vi "星际大战完整版.vi"() -> ()   [LabVIEW 2018]
panel:
  in  "关卡":dbl
  out "失败界面":picture
  out "胜利界面":picture
  out "敌机是否入侵":bool
  out "得分":dbl
  out "战舰爆炸":picture
  out "血量":dbl
  out "战舰血量":T1 scale=0.0..100.0
  out "敌机爆炸":picture
  in  "敌机数量":dbl
  in  "敌机速度":dbl
  out "敌机":picture
  out "按键":dbl
  out "战舰":T2
  out "激光武器1":T3
  out "激光武器 2":T3
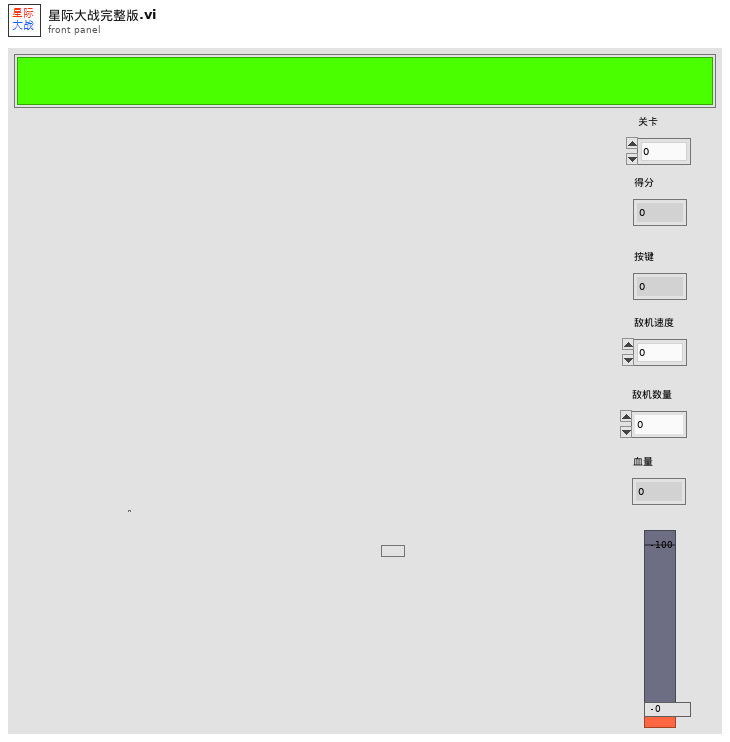
[diagram p1: front panel]
types:
  T1 = typedef "战列巡洋舰_血条.ctl" = dbl
  T2 = typedef "战列巡洋舰.ctl" = picture
  T3 = typedef "战列巡洋舰_激光武器.ctl" = picture
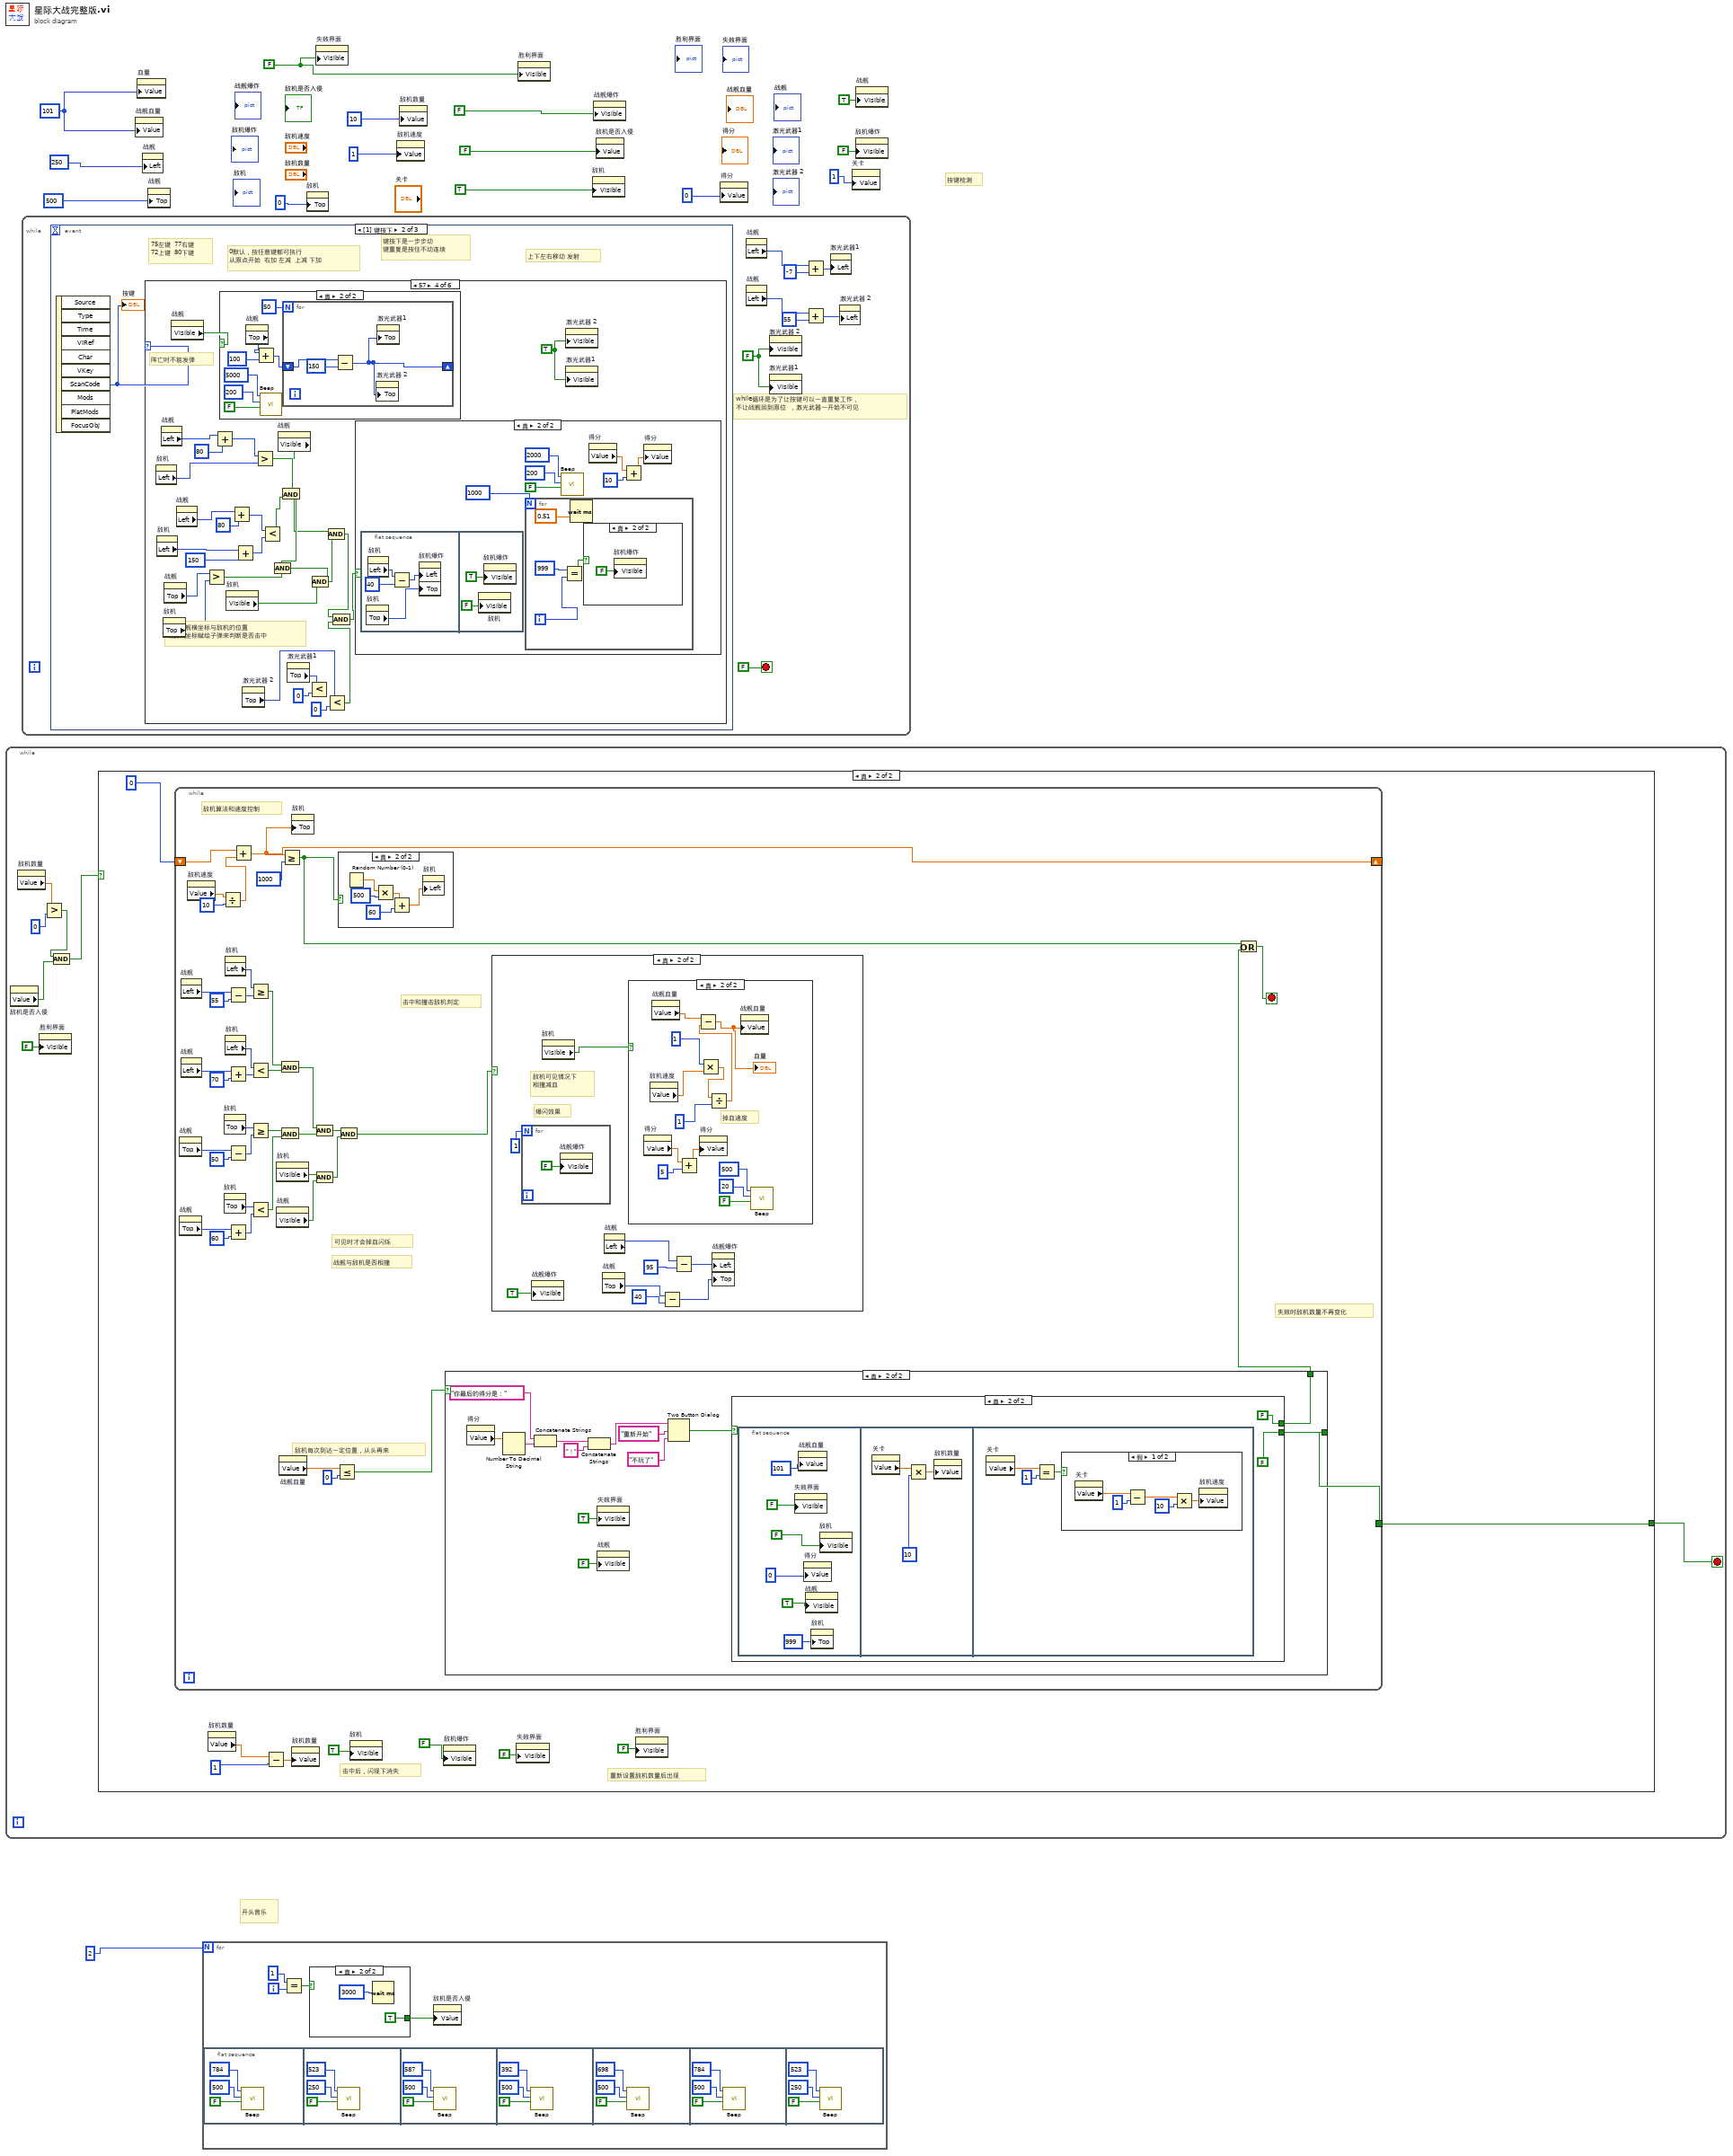
[diagram p0: block diagram]
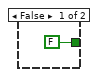
[diagram p2: hidden frame]
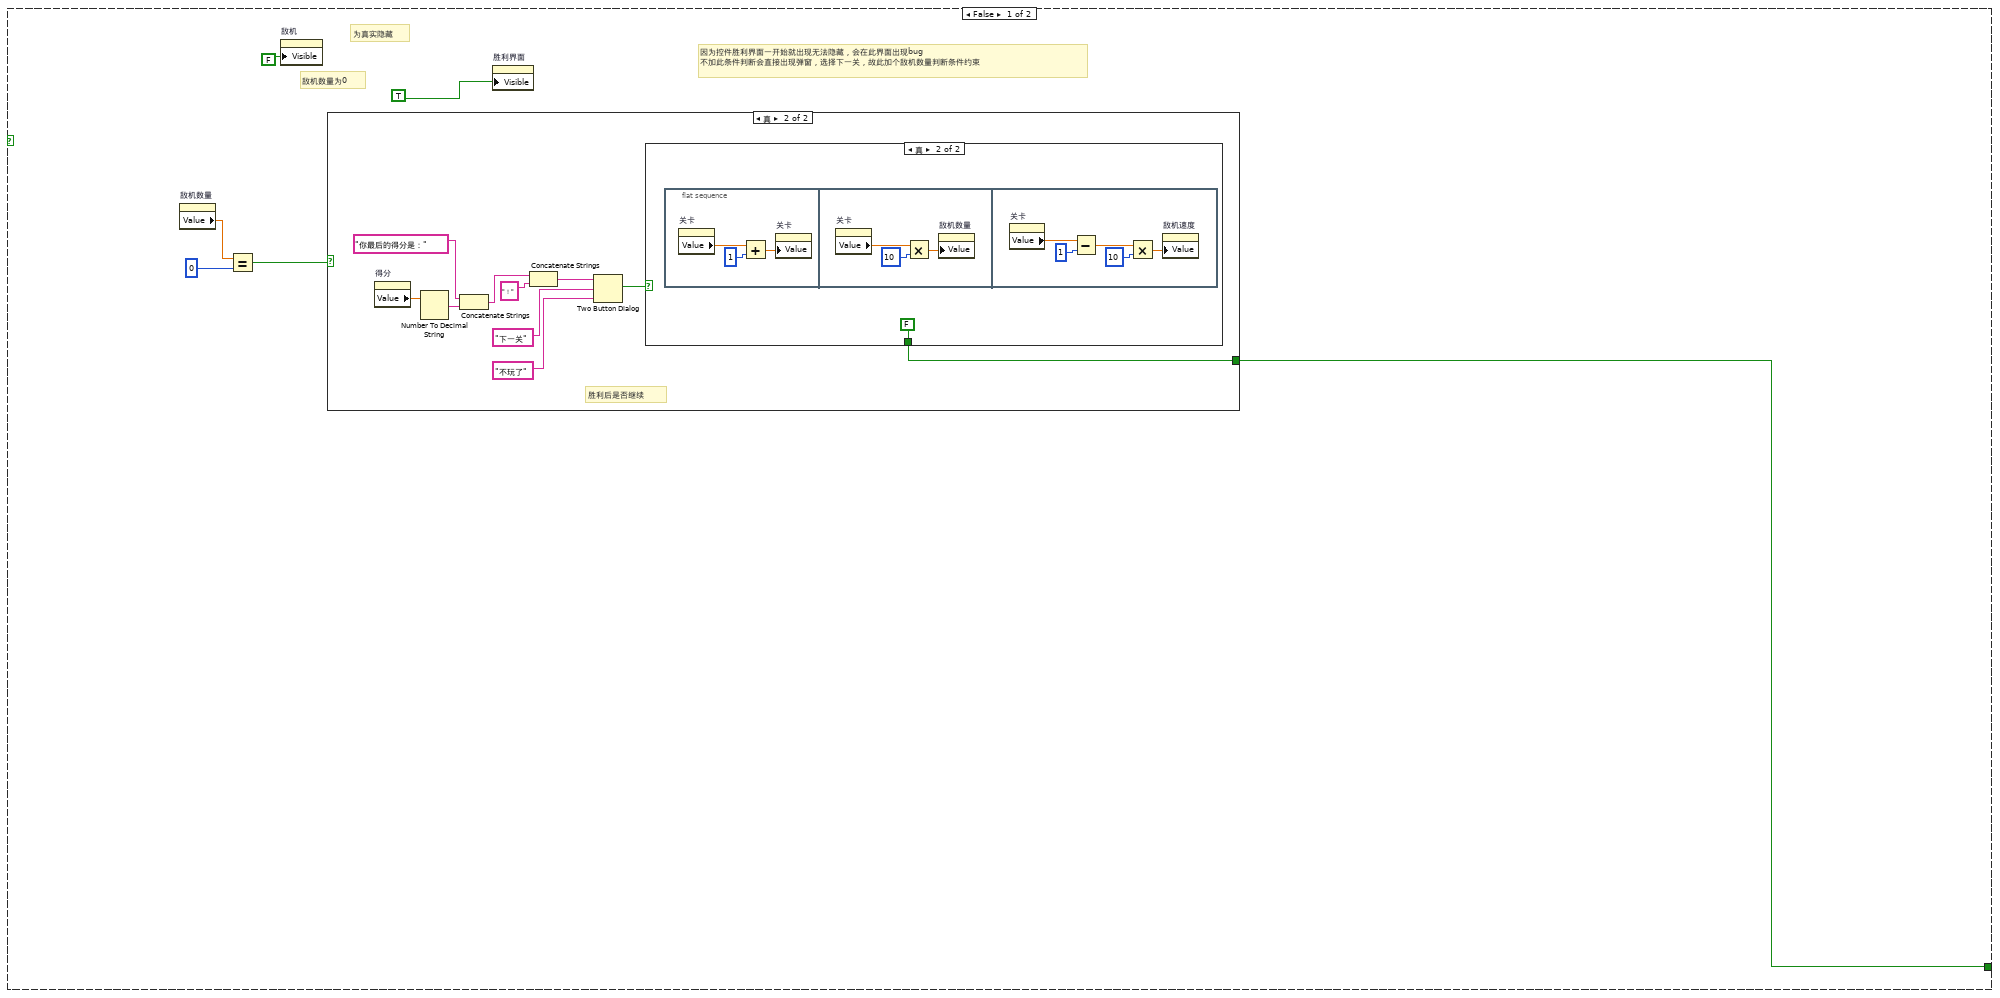
[diagram p3: hidden frame]
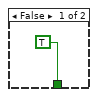
[diagram p5: hidden frame]
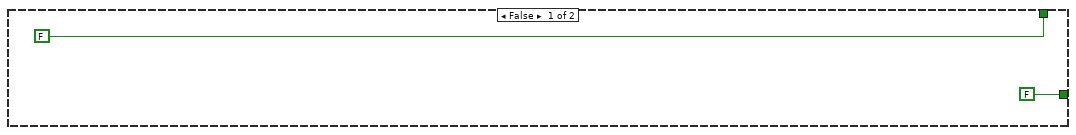
[diagram p6: hidden frame]
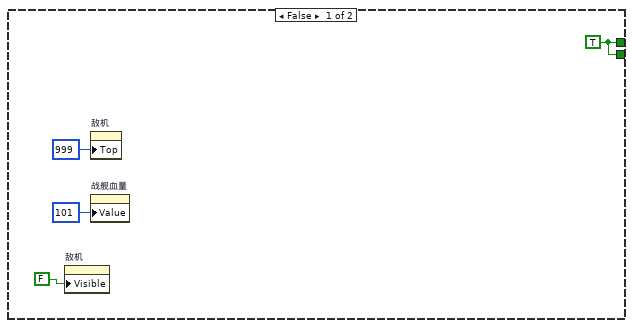
[diagram p7: hidden frame]
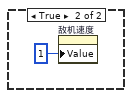
[diagram p8: hidden frame]
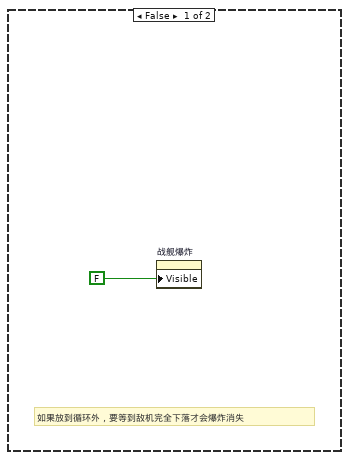
[diagram p9: hidden frame]
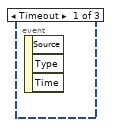
[diagram p12: hidden frame]
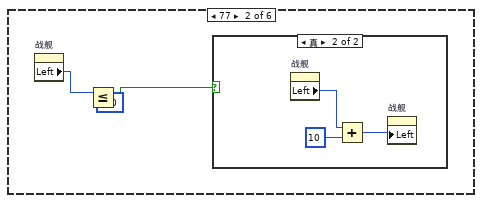
[diagram p14: hidden frame]
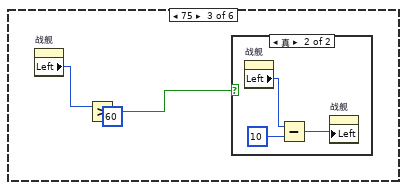
[diagram p16: hidden frame]
diagram:
  w1 = FALSE ("可见")
  w9 = 101
  # "开头音乐"
  # "按键检测"
  n1 = while {
    stop <- w17 stop-if-true
    n2 = property on="敌机是否入侵" class="Bool (严格)"() -> ("Value"=w20:bool)  [unwired: 2 in, 2 out]
    n3 = property on="敌机数量" class="DigNum (严格)"() -> ("Value"=w22:dbl)  [unwired: 2 in, 2 out]
    n4 = property on="胜利界面" class="Pict"("Visible"=FALSE ("可见")) -> ()  [unwired: 2 in, 2 out]
    n5 = Greater?(x=w22, y=0) -> (0:w19:bool)
    n6 = And(x=w19, y=w20) -> (x .and. y?=w18:bool)
    n7 = case shown="真" w18 {
      tunnel: [w26 w53] -> w17
      frame False {
        # "因为控件胜利界面一开始就出现无法隐藏，会在此界面出现bug\n不加此条件判断会直接出现弹窗，选择下一关，故此加个敌机数量判断条件约束"
        # "敌机数量为0"
        # "为真实隐藏"
        n8 = property on="敌机数量" class="DigNum (严格)"() -> ("Value"=w25:dbl)  [unwired: 2 in, 2 out]
        n9 = Equal?(x=w25, y=0) -> (x = y?=w23:bool)
        n10 = property on="敌机" class="Pict"("Visible"=FALSE ("可见")) -> ()  [unwired: 2 in, 2 out]
        n11 = case shown="真" w23 {
          tunnel: [_ w29] -> w26
          frame False {
          }
          frame True {
            # "胜利后是否继续"
            n12 = property on="得分" class="DigNum (严格)"() -> ("Value"=w37:dbl)  [unwired: 2 in, 2 out]
            n13 = Number To Decimal String(number=w37) -> (decimal integer string=w35:string)  [unwired: 1 in]
            n14 = Concatenate Strings("你最后的得分是：", w35) -> (w34:string)
            n15 = Concatenate Strings(w34, "！") -> (w32:string)
            n16 = Two Button Dialog(message=w32, 1:"不玩了" ("F按钮名称（“取消”）"), 2:"下一关" ("T按钮名称（“确定”）")) -> (T button?=w38:bool)
            n17 = case shown="真" w38 {
              tunnel: [TRUE FALSE] -> w29
              frame False {
              }
              frame True {
                n18 = flat-sequence {
                  frame #0 {
                    n19 = property on="关卡" class="DigNum (严格)"() -> ("Value"=w43:dbl)  [unwired: 2 in, 2 out]
                    n20 = Add(x=w43, y=1) -> (x+y=w41:dbl)
                    n21 = property on="关卡" class="DigNum (严格)"("Value"=w41) -> ()  [unwired: 2 in, 2 out]
                  }
                  frame #1 {
                    n22 = property on="关卡" class="DigNum (严格)"() -> ("Value"=w45:dbl)  [unwired: 2 in, 2 out]
                    n23 = Multiply(x=w45, y=10) -> (x*y=w46:dbl)
                    n24 = property on="敌机数量" class="DigNum (严格)"("Value"=w46) -> ()  [unwired: 2 in, 2 out]
                  }
                  frame #2 {
                    n25 = property on="关卡" class="DigNum (严格)"() -> ("Value"=w50:dbl)  [unwired: 2 in, 2 out]
                    n26 = Subtract(x=w50, y=1) -> (x-y=w48:dbl)
                    n27 = Multiply(x=w48, y=10) -> (x*y=w47:dbl)
                    n28 = property on="敌机速度" class="DigNum (严格)"("Value"=w47) -> ()  [unwired: 2 in, 2 out]
                  }
                }
              }
            }
          }
        }
        n29 = property on="胜利界面" class="Pict"("Visible"=TRUE ("可见")) -> ()  [unwired: 2 in, 2 out]
      }
      frame True {
        # "重新设置敌机数量后出现"
        # "击中后，闪现下消失"
        # "敌机每次到达一定位置，从头再来"
        n30 = while {
          shift-right: [w98] -> _
          shift-left: 0 -> [w100]
          tunnel: [w64] -> w53
          stop <- w62 stop-if-true
          # "失败时敌机数量不再变化"
          # "击中和撞击敌机判定"
          # "可见时才会掉血闪烁"
          # "战舰与敌机是否相撞"
          # "敌机算法和速度控制"
          n31 = property on="战舰" class="Pict (严格)"() -> ("Top"=w83:i32)  [unwired: 2 in, 2 out]
          n32 = property on="战舰" class="Pict (严格)"() -> ("Top"=w77:i32)  [unwired: 2 in, 2 out]
          n33 = property on="战舰" class="Pict (严格)"() -> ("Left"=w93:i32)  [unwired: 2 in, 2 out]
          n34 = property on="战舰" class="Pict (严格)"() -> ("Left"=w87:i32)  [unwired: 2 in, 2 out]
          n35 = property on="敌机速度" class="DigNum (严格)"() -> ("Value"=w97:dbl)  [unwired: 2 in, 2 out]
          n36 = Divide(x=w97, y=10) -> (x/y=w96:dbl)
          n37 = property on="敌机" class="Pict"() -> ("Top"=w84:i32)  [unwired: 2 in, 2 out]
          n38 = property on="敌机" class="Pict"() -> ("Top"=w76:i32)  [unwired: 2 in, 2 out]
          n39 = property on="敌机" class="Pict"() -> ("Left"=w94:i32)  [unwired: 2 in, 2 out]
          n40 = property on="敌机" class="Pict"() -> ("Left"=w89:i32)  [unwired: 2 in, 2 out]
          n41 = Subtract(x=w93, y=55) -> (x-y=w92:i32)
          n42 = Add(x=w87, y=70) -> (x+y=w86:i32)
          n43 = Subtract(x=w83, y=50) -> (x-y=w81:i32)
          n44 = Add(x=w77, y=60) -> (x+y=w79:i32)
          n45 = Add(x=w100, y=w96) -> (x+y=w98:dbl)
          n46 = Greater Or Equal?(x=w94, y=w92) -> (x >= y?=w90:bool)
          n47 = Less?(x=w89, y=w86) -> (x < y?=w85:bool)
          n48 = Greater Or Equal?(x=w84, y=w81) -> (x >= y?=w75:bool)
          n49 = Less?(x=w76, y=w79) -> (x < y?=w74:bool)
          n50 = property on="敌机" class="Pict"() -> ("Visible"=w67:bool)  [unwired: 2 in, 2 out]
          n51 = property on="战舰" class="Pict (严格)"() -> ("Visible"=w66:bool)  [unwired: 2 in, 2 out]
          n52 = And(x=w90, y=w85) -> (x .and. y?=w80:bool)
          n53 = And(x=w75, y=w74) -> (x .and. y?=w73:bool)
          n54 = property on="战舰血量" class="Slide (严格)"() -> ("Value"=w69:T1)  [unwired: 2 in, 2 out]
          n55 = Greater Or Equal?(x=w98, y=1000) -> (x >= y?=w63:bool)
          n56 = property on="敌机" class="Pict"("Top"=w98) -> ()  [unwired: 2 in, 2 out]
          n57 = And(x=w80, y=w73) -> (x .and. y?=w72:bool)
          n58 = And(x=w67, y=w66) -> (x .and. y?=w65:bool)
          n59 = Less Or Equal?(x=w69, y=0) -> (x <= y?=w70:bool)
          n60 = case shown="真" w63 {
            frame False {
            }
            frame True {
              n61 = Random Number (0-1)() -> (number: 0 to 1=w168:dbl)
              n62 = Multiply(x=w168, y=500) -> (x*y=w166:dbl)
              n63 = Add(x=w166, y=60) -> (x+y=w165:dbl)
              n64 = property on="敌机" class="Pict"("Left"=w165) -> ()  [unwired: 2 in, 2 out]
            }
          }
          n65 = And(x=w72, y=w65) -> (x .and. y?=w71:bool)
          n66 = case shown="真" w70 {
            tunnel: [FALSE w104] -> w64
            tunnel: [FALSE w103] -> w61
            frame False {
            }
            frame True {
              n67 = property on="得分" class="DigNum (严格)"() -> ("Value"=w115:dbl)  [unwired: 2 in, 2 out]
              n68 = Number To Decimal String(number=w115) -> (decimal integer string=w114:string)  [unwired: 1 in]
              n69 = Concatenate Strings("你最后的得分是：", w114) -> (w113:string)
              n70 = Concatenate Strings(w113, "！") -> (w112:string)
              n71 = property on="失败界面" class="Pict"("Visible"=TRUE ("可见")) -> ()  [unwired: 2 in, 2 out]
              n72 = property on="战舰" class="Pict (严格)"("Visible"=FALSE ("可见")) -> ()  [unwired: 2 in, 2 out]
              n73 = Two Button Dialog(message=w112, 1:"不玩了" ("F按钮名称（“取消”）"), 2:"重新开始" ("T按钮名称（“确定”）")) -> (T button?=w107:bool)
              n74 = case shown="真" w107 {
                tunnel: [w117 FALSE] -> w104
                tunnel: [w117 FALSE] -> w103
                frame False {
                  w117 = TRUE
                  n75 = property on="敌机" class="Pict"("Visible"=FALSE ("可见")) -> ()  [unwired: 2 in, 2 out]
                  n76 = property on="敌机" class="Pict"("Top"=999 ("位置:置顶")) -> ()  [unwired: 2 in, 2 out]
                  n77 = property on="战舰血量" class="Slide (严格)"("Value"=101) -> ()  [unwired: 2 in, 2 out]
                }
                frame True {
                  n78 = flat-sequence {
                    frame #0 {
                      n79 = property on="失败界面" class="Pict"("Visible"=FALSE ("可见")) -> ()  [unwired: 2 in, 2 out]
                      n80 = property on="战舰血量" class="Slide (严格)"("Value"=101) -> ()  [unwired: 2 in, 2 out]
                      n81 = property on="得分" class="DigNum (严格)"("Value"=0) -> ()  [unwired: 2 in, 2 out]
                      n82 = property on="战舰" class="Pict (严格)"("Visible"=TRUE ("可见")) -> ()  [unwired: 2 in, 2 out]
                      n83 = property on="敌机" class="Pict"("Top"=999 ("位置:置顶")) -> ()  [unwired: 2 in, 2 out]
                      n84 = property on="敌机" class="Pict"("Visible"=FALSE ("可见")) -> ()  [unwired: 2 in, 2 out]
                    }
                    frame #1 {
                      n85 = property on="关卡" class="DigNum (严格)"() -> ("Value"=w128:dbl)  [unwired: 2 in, 2 out]
                      n86 = Multiply(x=w128, y=10) -> (x*y=w130:dbl)
                      n87 = property on="敌机数量" class="DigNum (严格)"("Value"=w130) -> ()  [unwired: 2 in, 2 out]
                    }
                    frame #2 {
                      n88 = property on="关卡" class="DigNum (严格)"() -> ("Value"=w133:dbl)  [unwired: 2 in, 2 out]
                      n89 = Equal?(x=w133, y=1) -> (x = y?=w131:bool)
                      n90 = case shown="假" w131 {
                        frame False {
                          n91 = property on="关卡" class="DigNum (严格)"() -> ("Value"=w137:dbl)  [unwired: 2 in, 2 out]
                          n92 = Subtract(x=w137, y=1) -> (x-y=w134:dbl)
                          n93 = Multiply(x=w134, y=10) -> (x*y=w138:dbl)
                          n94 = property on="敌机速度" class="DigNum (严格)"("Value"=w138) -> ()  [unwired: 2 in, 2 out]
                        }
                        frame True {
                          n95 = property on="敌机速度" class="DigNum (严格)"("Value"=1) -> ()  [unwired: 2 in, 2 out]
                        }
                      }
                    }
                  }
                }
              }
            }
          }
          n96 = case shown="真" w71 {
            frame False {
              # "如果放到循环外，要等到敌机完全下落才会爆炸消失"
              n97 = property on="战舰爆炸" class="Pict"("Visible"=FALSE ("可见")) -> ()  [unwired: 2 in, 2 out]
            }
            frame True {
              # "爆闪效果"
              # "敌机可见情况下\n相撞减血"
              n98 = for {
                N: 1 -> [_]
                n99 = property on="战舰爆炸" class="Pict"("Visible"=FALSE ("可见")) -> ()  [unwired: 2 in, 2 out]
              }
              n100 = property on="战舰爆炸" class="Pict"("Visible"=TRUE ("可见")) -> ()  [unwired: 2 in, 2 out]
              n101 = property on="敌机" class="Pict"() -> ("Visible"=w149:bool)  [unwired: 2 in, 2 out]
              n102 = property on="战舰" class="Pict (严格)"() -> ("Top"=w144:i32)  [unwired: 2 in, 2 out]
              n103 = property on="战舰" class="Pict (严格)"() -> ("Left"=w147:i32)  [unwired: 2 in, 2 out]
              n104 = case shown="真" w149 {
                frame False {
                }
                frame True {
                  # "掉血速度"
                  n105 = property on="得分" class="DigNum (严格)"() -> ("Value"=w156:dbl)  [unwired: 2 in, 2 out]
                  n106 = property on="敌机速度" class="DigNum (严格)"() -> ("Value"=w162:dbl)  [unwired: 2 in, 2 out]
                  n107 = property on="战舰血量" class="Slide (严格)"() -> ("Value"=w163:T1)  [unwired: 2 in, 2 out]
                  n108 = Add(x=w156, y=5) -> (x+y=w155:dbl)
                  n109 = Multiply(x=1, y=w162) -> (x*y=w161:dbl)
                  n110 = property on="得分" class="DigNum (严格)"("Value"=w155) -> ()  [unwired: 2 in, 2 out]
                  n111 = Divide(x=w161, y=1) -> (x/y=w158:dbl)
                  n112 = Subtract(x=w163, y=w158) -> (x-y=w157:T1)
                  "血量" <- w157
                  n113 = property on="战舰血量" class="Slide (严格)"("Value"=w157) -> ()  [unwired: 2 in, 2 out]
                  n114 = call <vilib>:"Beep.vi"("use system alert? (T)"=FALSE, "duration (msec)"=u32 20, "frequency (Hz)"=u32 500) -> ()  [unwired: 9 in]
                }
              }
              n115 = Subtract(x=w144, y=40) -> (x-y=w142:i32)
              n116 = Subtract(x=w147, y=95) -> (x-y=w145:i32)
              n117 = property on="战舰爆炸" class="Pict"("Left"=w145, "Top"=w142) -> ()  [unwired: 2 in, 2 out]
            }
          }
          n118 = Or(x=w63, y=w61) -> (x .or. y?=w62:bool)
        }
        n119 = property on="敌机数量" class="DigNum (严格)"() -> ("Value"=w58:dbl)  [unwired: 2 in, 2 out]
        n120 = Subtract(x=w58, y=1) -> (x-y=w59:dbl)
        n121 = property on="敌机数量" class="DigNum (严格)"("Value"=w59) -> ()  [unwired: 2 in, 2 out]
        n122 = property on="敌机" class="Pict"("Visible"=TRUE ("可见")) -> ()  [unwired: 2 in, 2 out]
        n123 = property on="敌机爆炸" class="Pict"("Visible"=FALSE ("可见")) -> ()  [unwired: 2 in, 2 out]
        n124 = property on="失败界面" class="Pict"("Visible"=FALSE ("可见")) -> ()  [unwired: 2 in, 2 out]
        n125 = property on="胜利界面" class="Pict"("Visible"=FALSE ("可见")) -> ()  [unwired: 2 in, 2 out]
      }
    }
  }
  n126 = while {
    stop <- FALSE stop-if-true
    w169 = FALSE
    # "while循环是为了让按键可以一直重复工作，\n不让战舰回到原位  ，激光武器一开始不可见"
    n127 = event shown="[1] 键按下" {
      selector: _ -> [_ _ _]
      dyn-events: _ -> [_ _ _]
      timeout: _ -> [_ _ _]
      event Timeout {
        n128 = event-data() -> ()  [unwired: 1 in, 3 out]
      }
      event Key Down {
        # "上下左右移动 发射"
        # "键按下是一步步动\n键重复是按住不动连续"
        # "75左键  77右键\n72上键  80下键"
        # "0默认，按任意键都可执行\n从原点开始  右加 左减  上减 下加"
        n129 = event-data() -> ("ScanCode"=w177:i16)  [unwired: 1 in, 9 out]
        "按键" <- w177
        n130 = case shown="57" w177 {
          frame 0, Default {
          }
          frame 77 {
            n131 = property on="战舰" class="Pict (严格)"() -> ("Left"=w180:i32)  [unwired: 2 in, 2 out]
            n132 = Less Or Equal?(x=w180, y=500) -> (x <= y?=w178:bool)
            n133 = case shown="真" w178 {
              frame False {
              }
              frame True {
                n134 = property on="战舰" class="Pict (严格)"() -> ("Left"=w182:i32)  [unwired: 2 in, 2 out]
                n135 = Add(x=w182, y=10) -> (x+y=w183:i32)
                n136 = property on="战舰" class="Pict (严格)"("Left"=w183) -> ()  [unwired: 2 in, 2 out]
              }
            }
          }
          frame 75 {
            n137 = property on="战舰" class="Pict (严格)"() -> ("Left"=w186:i32)  [unwired: 2 in, 2 out]
            n138 = Greater?(x=w186, y=60) -> (0:w184:bool)
            n139 = case shown="真" w184 {
              frame False {
              }
              frame True {
                n140 = property on="战舰" class="Pict (严格)"() -> ("Left"=w188:i32)  [unwired: 2 in, 2 out]
                n141 = Subtract(x=w188, y=10) -> (x-y=w189:i32)
                n142 = property on="战舰" class="Pict (严格)"("Left"=w189) -> ()  [unwired: 2 in, 2 out]
              }
            }
          }
          frame 57 {
            w218 = TRUE
            # "阵亡时不能发弹"
            # "判断战舰横坐标与敌机的位置\n战舰纵坐标赋给子弹来判断是否击中"
            n143 = property on="敌机" class="Pict"() -> ("Left"=w215:i32)  [unwired: 2 in, 2 out]
            n144 = property on="敌机" class="Pict"() -> ("Left"=w208:i32)  [unwired: 2 in, 2 out]
            n145 = property on="战舰" class="Pict (严格)"() -> ("Left"=w217:i32)  [unwired: 2 in, 2 out]
            n146 = property on="敌机" class="Pict"() -> ("Top"=w202:i32)  [unwired: 2 in, 2 out]
            n147 = property on="战舰" class="Pict (严格)"() -> ("Top"=w203:i32)  [unwired: 2 in, 2 out]
            n148 = property on="战舰" class="Pict (严格)"() -> ("Visible"=w197:bool)  [unwired: 2 in, 2 out]
            n149 = property on="战舰" class="Pict (严格)"() -> ("Left"=w210:i32)  [unwired: 2 in, 2 out]
            n150 = Greater?(x=w203, y=w202) -> (0:w204:bool)
            n151 = Add(x=w217, y=80) -> (x+y=w214:i32)
            n152 = case shown="真" w197 {
              frame False {
              }
              frame True {
                n153 = property on="战舰" class="Pict (严格)"() -> ("Top"=w224:i32)  [unwired: 2 in, 2 out]
                n154 = Add(x=w224, y=100) -> (x+y=w222:i32)
                n155 = call <vilib>:"Beep.vi"("use system alert? (T)"=FALSE, "duration (msec)"=u32 200, "frequency (Hz)"=u32 5000) -> ()  [unwired: 9 in]
                n156 = for {
                  N: 50 -> [_]
                  shift-right: [w226] -> _
                  shift-left: w222 -> [w228]
                  n157 = Subtract(x=w228, y=150) -> (x-y=w226:i32)
                  n158 = property on="激光武器 2" class="Pict (严格)"("Top"=w226) -> ()  [unwired: 2 in, 2 out]
                  n159 = property on="激光武器1" class="Pict (严格)"("Top"=w226) -> ()  [unwired: 2 in, 2 out]
                }
              }
            }
            n160 = property on="敌机" class="Pict"() -> ("Visible"=w200:bool)  [unwired: 2 in, 2 out]
            n161 = Add(x=w210, y=80) -> (x+y=w212:i32)
            n162 = Add(x=w208, y=150) -> (x+y=w207:i32)
            n163 = property on="激光武器 2" class="Pict (严格)"() -> ("Top"=w193:i32)  [unwired: 2 in, 2 out]
            n164 = Greater?(x=w214, y=w215) -> (0:w213:bool)
            n165 = Less?(x=w212, y=w207) -> (x < y?=w209:bool)
            n166 = property on="战舰" class="Pict (严格)"() -> ("Visible"=w199:bool)  [unwired: 2 in, 2 out]
            n167 = And(x=w213, y=w209) -> (x .and. y?=w205:bool)
            n168 = And(x=w205, y=w204) -> (x .and. y?=w201:bool)
            n169 = property on="激光武器1" class="Pict (严格)"() -> ("Top"=w195:i32)  [unwired: 2 in, 2 out]
            n170 = Less?(x=w195, y=0) -> ()  [unwired: 1 out]
            n171 = And(x=w201, y=w200) -> (x .and. y?=w198:bool)
            n172 = And(x=w199, y=w198) -> (x .and. y?=w191:bool)
            n173 = Less?(x=w193, y=0) -> (x < y?=w192:bool)
            n174 = And(x=w191, y=w192) -> (x .and. y?=w190:bool)
            n175 = case shown="真" w190 {
              frame False {
              }
              frame True {
                n176 = flat-sequence {
                  frame #0 {
                    n177 = property on="敌机" class="Pict"() -> ("Top"=w239:i32)  [unwired: 2 in, 2 out]
                    n178 = property on="敌机" class="Pict"() -> ("Left"=w237:i32)  [unwired: 2 in, 2 out]
                    n179 = Subtract(x=w237, y=40) -> (x-y=w236:i32)
                    n180 = property on="敌机爆炸" class="Pict"("Left"=w236, "Top"=w239) -> ()  [unwired: 2 in, 2 out]
                  }
                  frame #1 {
                    n181 = property on="敌机" class="Pict"("Visible"=FALSE ("可见")) -> ()  [unwired: 2 in, 2 out]
                    n182 = property on="敌机爆炸" class="Pict"("Visible"=TRUE ("可见")) -> ()  [unwired: 2 in, 2 out]
                  }
                }
                n183 = for {
                  N: 1000 -> [_]
                  i -> [w244]
                  n184 = Equal?(x=999, y=w244) -> (x = y?=w245:bool)
                  n185 = Wait (ms)(milliseconds to wait=0.51) -> ()  [unwired: 1 out]
                  n186 = case shown="真" w245 {
                    frame False {
                    }
                    frame True {
                      n187 = property on="敌机爆炸" class="Pict"("Visible"=FALSE ("可见")) -> ()  [unwired: 2 in, 2 out]
                    }
                  }
                }
                n188 = call <vilib>:"Beep.vi"("use system alert? (T)"=FALSE, "duration (msec)"=u32 200, "frequency (Hz)"=u32 2000) -> ()  [unwired: 9 in]
                n189 = property on="得分" class="DigNum (严格)"() -> ("Value"=w234:dbl)  [unwired: 2 in, 2 out]
                n190 = Add(x=w234, y=10) -> (x+y=w232:dbl)
                n191 = property on="得分" class="DigNum (严格)"("Value"=w232) -> ()  [unwired: 2 in, 2 out]
              }
            }
            n192 = property on="激光武器 2" class="Pict (严格)"("Visible"=w218) -> ()  [unwired: 2 in, 2 out]
            n193 = property on="激光武器1" class="Pict (严格)"("Visible"=w218) -> ()  [unwired: 2 in, 2 out]
          }
          frame 80 {
            n194 = property on="战舰" class="Pict (严格)"() -> ("Top"=w249:i32)  [unwired: 2 in, 2 out]
            n195 = Less?(x=w249, y=525) -> (x < y?=w247:bool)
            n196 = case shown="真" w247 {
              frame False {
              }
              frame True {
                n197 = property on="战舰" class="Pict (严格)"() -> ("Top"=w251:i32)  [unwired: 2 in, 2 out]
                n198 = Add(x=w251, y=10) -> (x+y=w250:i32)
                n199 = property on="战舰" class="Pict (严格)"("Top"=w250) -> ()  [unwired: 2 in, 2 out]
              }
            }
          }
          frame 72 {
            n200 = property on="战舰" class="Pict (严格)"() -> ("Top"=w255:i32)  [unwired: 2 in, 2 out]
            n201 = Greater Or Equal?(x=w255, y=25) -> (x >= y?=w254:bool)
            n202 = case shown="真" w254 {
              frame False {
              }
              frame True {
                n203 = property on="战舰" class="Pict (严格)"() -> ("Top"=w258:i32)  [unwired: 2 in, 2 out]
                n204 = Subtract(x=w258, y=10) -> (x-y=w257:i32)
                n205 = property on="战舰" class="Pict (严格)"("Top"=w257) -> ()  [unwired: 2 in, 2 out]
              }
            }
          }
        }
      }
      event Key Repeat {
        # "75左键  77右键\n72上键  80下键\n空格 57"
        # "0默认，按任意键都可执行\n从原点开始  右加 左减  上减 下加"
        n206 = event-data() -> ("ScanCode"=w259:i16)  [unwired: 1 in, 9 out]
        n207 = case shown="72" w259 {
          frame 0, Default {
          }
          frame 77 {
            n208 = property on="战舰" class="Pict (严格)"() -> ("Left"=w262:i32)  [unwired: 2 in, 2 out]
            n209 = Less Or Equal?(x=w262, y=500) -> (x <= y?=w261:bool)
            n210 = case shown="真" w261 {
              frame False {
              }
              frame True {
                n211 = property on="战舰" class="Pict (严格)"() -> ("Left"=w264:i32)  [unwired: 2 in, 2 out]
                n212 = Add(x=w264, y=10) -> (x+y=w265:i32)
                n213 = property on="战舰" class="Pict (严格)"("Left"=w265) -> ()  [unwired: 2 in, 2 out]
              }
            }
          }
          frame 75 {
            n214 = property on="战舰" class="Pict (严格)"() -> ("Left"=w268:i32)  [unwired: 2 in, 2 out]
            n215 = Greater Or Equal?(x=w268, y=25) -> (x >= y?=w267:bool)
            n216 = case shown="真" w267 {
              frame False {
              }
              frame True {
                n217 = property on="战舰" class="Pict (严格)"() -> ("Left"=w271:i32)  [unwired: 2 in, 2 out]
                n218 = Subtract(x=w271, y=10) -> (x-y=w270:i32)
                n219 = property on="战舰" class="Pict (严格)"("Left"=w270) -> ()  [unwired: 2 in, 2 out]
              }
            }
          }
          frame 80 {
            n220 = property on="战舰" class="Pict (严格)"() -> ("Top"=w274:i32)  [unwired: 2 in, 2 out]
            n221 = Less Or Equal?(x=w274, y=525) -> (x <= y?=w273:bool)
            n222 = case shown="真" w273 {
              frame False {
              }
              frame True {
                n223 = property on="战舰" class="Pict (严格)"() -> ("Top"=w276:i32)  [unwired: 2 in, 2 out]
                n224 = Add(x=w276, y=10) -> (x+y=w275:i32)
                n225 = property on="战舰" class="Pict (严格)"("Top"=w275) -> ()  [unwired: 2 in, 2 out]
              }
            }
          }
          frame 72 {
            n226 = property on="战舰" class="Pict (严格)"() -> ("Top"=w280:i32)  [unwired: 2 in, 2 out]
            n227 = Greater Or Equal?(x=w280, y=25) -> (x >= y?=w279:bool)
            n228 = case shown="真" w279 {
              frame False {
              }
              frame True {
                n229 = property on="战舰" class="Pict (严格)"() -> ("Top"=w283:i32)  [unwired: 2 in, 2 out]
                n230 = Subtract(x=w283, y=10) -> (x-y=w282:i32)
                n231 = property on="战舰" class="Pict (严格)"("Top"=w282) -> ()  [unwired: 2 in, 2 out]
              }
            }
          }
        }
      }
    }
    n232 = property on="战舰" class="Pict (严格)"() -> ("Left"=w175:i32)  [unwired: 2 in, 2 out]
    n233 = property on="战舰" class="Pict (严格)"() -> ("Left"=w171:i32)  [unwired: 2 in, 2 out]
    n234 = property on="激光武器 2" class="Pict (严格)"("Visible"=w169) -> ()  [unwired: 2 in, 2 out]
    n235 = property on="激光武器1" class="Pict (严格)"("Visible"=w169) -> ()  [unwired: 2 in, 2 out]
    n236 = Add(x=w175, y=-7) -> (x+y=w174:i32)
    n237 = Add(x=w171, y=55) -> (x+y=w170:i32)
    n238 = property on="激光武器1" class="Pict (严格)"("Left"=w174) -> ()  [unwired: 2 in, 2 out]
    n239 = property on="激光武器 2" class="Pict (严格)"("Left"=w170) -> ()  [unwired: 2 in, 2 out]
  }
  n240 = property on="战舰血量" class="Slide (严格)"("Value"=w9) -> ()  [unwired: 2 in, 2 out]
  n241 = property on="血量" class="DigNum (严格)"("Value"=w9) -> ()  [unwired: 2 in, 2 out]
  n242 = property on="战舰" class="Pict (严格)"("Left"=250 ("位置:居左")) -> ()  [unwired: 2 in, 2 out]
  n243 = property on="战舰" class="Pict (严格)"("Top"=500 ("位置:置顶")) -> ()  [unwired: 2 in, 2 out]
  n244 = for {
    N: 2 -> [_]
    i -> [w285]
    n245 = flat-sequence {
      frame #0 {
        n246 = call <vilib>:"Beep.vi"("use system alert? (T)"=FALSE, "duration (msec)"=500, "frequency (Hz)"=784) -> ()  [unwired: 9 in]
      }
      frame #1 {
        n247 = call <vilib>:"Beep.vi"("use system alert? (T)"=FALSE, "duration (msec)"=250, "frequency (Hz)"=523) -> ()  [unwired: 9 in]
      }
      frame #2 {
        n248 = call <vilib>:"Beep.vi"("use system alert? (T)"=FALSE, "duration (msec)"=500, "frequency (Hz)"=587) -> ()  [unwired: 9 in]
      }
      frame #3 {
        n249 = call <vilib>:"Beep.vi"("use system alert? (T)"=FALSE, "duration (msec)"=500, "frequency (Hz)"=392) -> ()  [unwired: 9 in]
      }
      frame #4 {
        n250 = call <vilib>:"Beep.vi"("use system alert? (T)"=FALSE, "duration (msec)"=500, "frequency (Hz)"=698) -> ()  [unwired: 9 in]
      }
      frame #5 {
        n251 = call <vilib>:"Beep.vi"("use system alert? (T)"=FALSE, "duration (msec)"=500, "frequency (Hz)"=784) -> ()  [unwired: 9 in]
      }
      frame #6 {
        n252 = call <vilib>:"Beep.vi"("use system alert? (T)"=FALSE, "duration (msec)"=250, "frequency (Hz)"=523) -> ()  [unwired: 9 in]
      }
    }
    n253 = Equal?(x=1, y=w285) -> (x = y?=w287:bool)
    n254 = case shown="真" w287 {
      tunnel: [FALSE ("敌机是否入侵") TRUE ("敌机是否入侵")] -> w284
      frame False {
      }
      frame True {
        n255 = Wait (ms)(milliseconds to wait=u32 3000 ("等待时间（毫秒）")) -> ()  [unwired: 1 out]
      }
    }
    n256 = property on="敌机是否入侵" class="Bool (严格)"("Value"=w284) -> ()  [unwired: 2 in, 2 out]
  }
  n257 = property on="敌机" class="Pict"("Top"=0) -> ()  [unwired: 2 in, 2 out]
  n258 = property on="失败界面" class="Pict"("Visible"=w1) -> ()  [unwired: 2 in, 2 out]
  n259 = property on="敌机速度" class="DigNum (严格)"("Value"=1) -> ()  [unwired: 2 in, 2 out]
  n260 = property on="敌机数量" class="DigNum (严格)"("Value"=10) -> ()  [unwired: 2 in, 2 out]
  n261 = property on="胜利界面" class="Pict"("Visible"=w1) -> ()  [unwired: 2 in, 2 out]
  n262 = property on="敌机" class="Pict"("Visible"=TRUE ("可见")) -> ()  [unwired: 2 in, 2 out]
  n263 = property on="战舰爆炸" class="Pict"("Visible"=FALSE ("可见")) -> ()  [unwired: 2 in, 2 out]
  n264 = property on="敌机是否入侵" class="Bool (严格)"("Value"=FALSE ("敌机是否入侵")) -> ()  [unwired: 2 in, 2 out]
  n265 = property on="得分" class="DigNum (严格)"("Value"=0) -> ()  [unwired: 2 in, 2 out]
  n266 = property on="关卡" class="DigNum (严格)"("Value"=1) -> ()  [unwired: 2 in, 2 out]
  n267 = property on="敌机爆炸" class="Pict"("Visible"=FALSE ("可见")) -> ()  [unwired: 2 in, 2 out]
  n268 = property on="战舰" class="Pict (严格)"("Visible"=TRUE ("可见")) -> ()  [unwired: 2 in, 2 out]
